vi "Autonomous Independent.vi"   [LabVIEW 2013]
doc: "This VI is called when autonomous begins, and will automatically be terminated when autonomous ends. You can carry out timed or sensor driven robot movement independently without needing to return to the caller."
uses:
  <vilib>/Rock Robotics/WPI/Solenoid/WPI_SolenoidValue.ctl
  Robot Global Data.vi
  <vilib>/Rock Robotics/WPI/Solenoid/WPI_SolenoidSetEnum.vi
  <vilib>/Rock Robotics/WPI/RobotDrive/WPI_RobotDriveArcadeDrive_Standard(NoSaturation).vi
  <vilib>/Rock Robotics/WPI/RobotDrive/WPI_RobotDriveGetSetRefNum.vi
  <vilib>/Rock Robotics/WPI/Joystick/WPI_JoystickGetSetRefNum.vi
panel:
  # "Be sure to right-click and choose Data Operations>>Make Current Value default if you want to save the array values with the VI"
types:
  T1 = typedef "WPI_JoystickDevRef.ctl" = cluster{"Device":T2}
  T2 = typedef "WPI_JoystickDeviceEnum.ctl" = enum16{"USB 1", "USB 2", "USB 3", "USB 4", "Kinect 1", "Kinect 2"}
  T3 = cluster{"axis 1 (x)":dbl, "axis 2 (y)":dbl, "axis 3 (throttle)":dbl, "axis 4":dbl, "axis 5":dbl, "axis 6":dbl}
  T4 = typedef "WPI_SolenoidValue.ctl" = enum16{"Off", "On", "Forward", "Reverse"}
  T5 = typedef "WPI_SolenoidDevRef.ctl" = cluster{"DevStatus":errorcluster, "Solenoid Module":T6, "Forward Solenoid Channel":T7, "Reverse Solenoid Channel":T7}
  T6 = typedef "FPGA_TypedefSolenoidModule.ctl" = enum16{"Solenoid Module 1", "Solenoid Module 2"}
  T7 = typedef "WPI_SolenoidChannel.ctl" = enum8{"Solenoid 1", "Solenoid 2", "Solenoid 3", "Solenoid 4", "Solenoid 5", "Solenoid 6", "Solenoid 7", "Solenoid 8", "Invalid"}
  T8 = typedef "WPI_RobotDriveDevRef.ctl" = cluster{"DevStatus":errorcluster, "Motors[]":T9[], "Square Inputs":bool, "Max Output":dbl, "Isochronous":bool}
  T9 = typedef "WPI_MotorControlDeviceRef.ctl" = cluster{"DeviceStatus":errorcluster, "Type":enum16{"PWM", "CAN"}, "PWM":cluster{"Digital Module":T10, "PWM Channel":T11, "DeadBand":T12}, "CAN":cluster{"Device Number":u8, "Control Mode":T13, "Semaphore":T14, "Max Vout":dbl}, "Invert":bool, "TransformRef":T15, "InvTransformRef":T15}
  T10 = typedef "FPGA_TypedefDigitalModule.ctl" = enum16{"Digital Module 1", "Digital Module 2"}
  T11 = typedef "FPGA_DIOPWMChannel.ctl" = enum8{"PWM 1", "PWM 2", "PWM 3", "PWM 4", "PWM 5", "PWM 6", "PWM 7", "PWM 8", "PWM 9", "PWM 10", "Invalid"}
  T12 = typedef "WPI_PWMDeadband.ctl" = cluster{"Name":string, "maxPositivePwm":i32, "minPositivePwm":i32, "centerPwm":i32, "maxNegativePwm":i32, "minNegativePwm":i32, "angularRange":u16}
  T13 = typedef "WPI_CANJaguar_ControlMode.ctl" = enum8{"Percent VBus", "Current", "Speed", "Position", "Voltage"}
  T14 = typedef "Semaphore RefNum" = refnum<k1>
  T15 = typedef "WPI_PWMTransform_ConPane.ctl" = refnum<vi>
  T16 = typedef "TargetType.ctl" = enum16{"Not Hot", "Hot"}
  T17 = cluster{"Distance (ft)":dbl, "Target Center (-1 to 1)":cluster{"X":dbl, "Y":dbl}, "Left":bool, "State":T16}[]
  T18 = cluster{"Distance (ft)":dbl, "Target Center (-1 to 1)":cluster{"X":dbl, "Y":dbl}, "Left":bool, "State":T16}
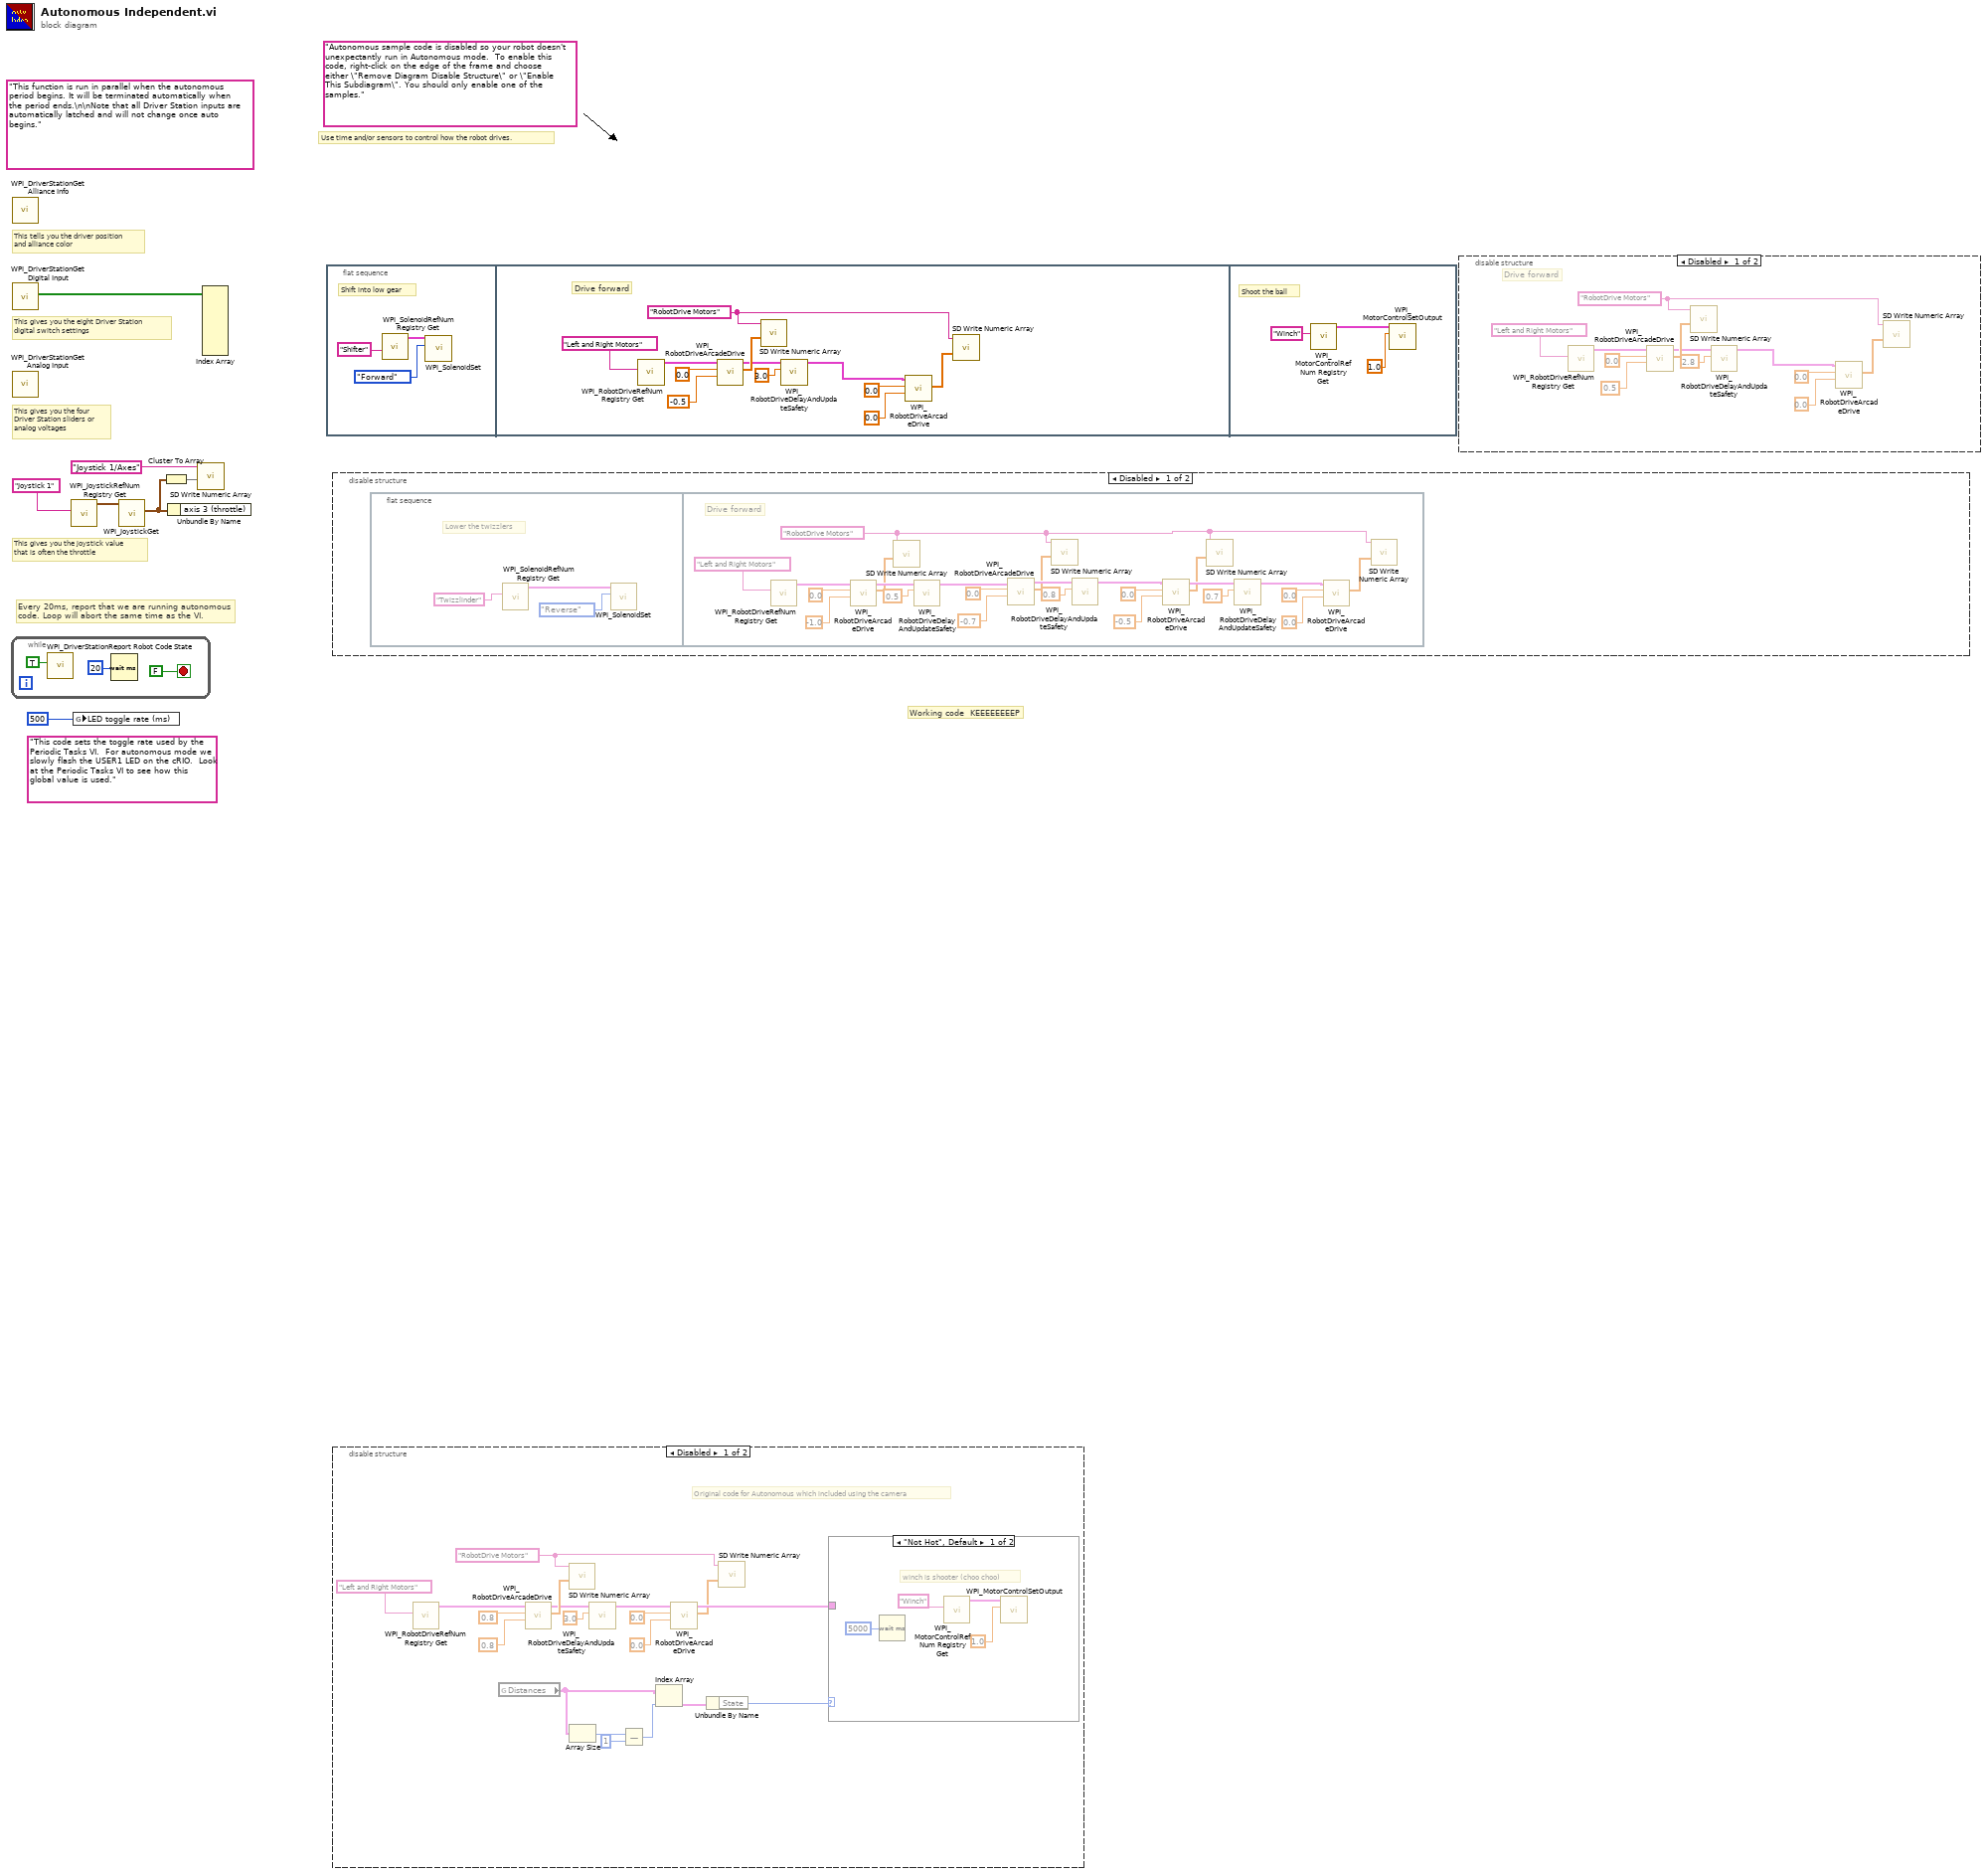
[diagram p0: block diagram]
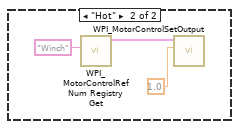
[diagram p4: hidden frame]
diagram:
  (unwired) "This code sets the toggle rate used by the Periodic Tasks VI.  For autonomous mode we slowly flash the USER1 LED on the cRIO.  Look at the Periodic Tasks VI to see how this global value is used."
  (unwired) "Autonomous sample code is disabled so your robot doesn't unexpectantly run in Autonomous mode.  To enable this code, right-click on the edge of the frame and choose either \"Remove Diagram Disable Structure\" or \"Enable This Subdiagram\". You should only enable one of the samples."
  (unwired) "This function is run in parallel when the autonomous period begins. It will be terminated automatically when the period ends.\n\nNote that all Driver Station inputs are automatically latched and will not change once auto begins."
  # "Working code  KEEEEEEEEP"
  # "Every 20ms, report that we are running autonomous\ncode. Loop will abort the same time as the VI."
  # "This gives you the joystick value\nthat is often the throttle"
  # "Use time and/or sensors to control how the robot drives."
  # "This tells you the driver position\nand alliance color"
  # "This gives you the eight Driver Station\ndigital switch settings"
  # "This gives you the four\nDriver Station sliders or\nanalog voltages"
  n1 = while {
    stop <- FALSE stop-if-true
    n2 = call <vilib>:"WPI_DriverStationReport Robot Code State.vi"("Autonomous"=TRUE) -> ()  [unwired: 10 in, 1 out]
    n3 = Wait (ms)(milliseconds to wait=u32 20) -> ()  [unwired: 1 out]
  }
  n4 = call <vilib>:"WPI_DriverStationGet Alliance Info.vi"() -> ()  [unwired: 12 out]
  n5 = call <vilib>:"WPI_DriverStationGet Digital Input.vi"() -> ("Driver Station Digital Input (1-8)"=w7:bool[])  [unwired: 11 out]
  n6 = call <vilib>:"WPI_DriverStationGet Analog Input.vi"() -> ()  [unwired: 12 out]
  n7 = call <vilib>:"WPI_JoystickRefNum Registry Get.vi"("refnum name"="Joystick 1") -> ("JoystickDevRef"=w5:T1)  [unwired: 1 in, 9 out]
  n8 = global write "Robot Global Data.vi" "LED toggle rate (ms)"(u32 500 ("LED ms toggle rate")) -> ()
  n9 = call <vilib>:"WPI_JoystickGet.vi"("JoystickDevRef"=w5) -> ("Axes"=w2:T3)  [unwired: 1 in, 5 out]
  n10 = Cluster To Array(cluster=w2) -> (array=w3:dbl[])
  n11 = Unbundle By Name(w2) -> ()  [unwired: 1 out]
  n12 = call <vilib>:"SD Write Numeric Array.vi"("Numeric Array"=w3, "Name"="Joystick 1/Axes") -> ()  [unwired: 8 in, 2 out]
  n13 = Index Array(array=w7) -> ()  [unwired: 8 in, 8 out]
  n14 = flat-sequence {
    frame #0 {
      # "Shift into low gear"
      n15 = call <vilib>:"WPI_SolenoidRefNum Registry Get.vi"("refnum name"="Shifter") -> ("SolenoidDevRef"=w12:T5)  [unwired: 9 in, 1 out]
      n16 = call-poly <vilib>:"WPI_SolenoidSet.vi"("Value"=WPI_SolenoidValue."Forward", "SolenoidDevRef"=w12) -> ()  [unwired: 1 in, 9 out]
    }
    frame #1 {
      w15 = "RobotDrive Motors" ("Name")
      # "Drive forward"
      n17 = call <vilib>:"WPI_RobotDriveRefNum Registry Get.vi"("refnum name"="Left and Right Motors") -> ("RobotDriveDevRef"=w24:T8)  [unwired: 1 in, 9 out]
      n18 = call-poly <vilib>:"WPI_RobotDriveArcadeDrive.vi"("Y axis value"=-0.5 ("X axis value"), "X axis value"=0.0, "RobotDriveDevRef"=w24) -> ("Motor Values"=w25:dbl[], "RobotDriveDevRef"=w21:T8)  [unwired: 1 in, 6 out]
      n19 = call <vilib>:"SD Write Numeric Array.vi"("Numeric Array"=w25, "Name"=w15) -> ()  [unwired: 8 in, 2 out]
      n20 = call <vilib>:"WPI_RobotDriveDelayAndUpdateSafety.vi"("Delay (s)"=3.0, "RobotDriveDevRef"=w21) -> ("RobotDriveDevRef 2"=w14:T8)  [unwired: 8 in, 1 out]
      n21 = call-poly <vilib>:"WPI_RobotDriveArcadeDrive.vi"("Y axis value"=0.0 ("X axis value"), "X axis value"=0.0, "RobotDriveDevRef"=w14) -> ("Motor Values"=w18:dbl[])  [unwired: 1 in, 7 out]
      n22 = call <vilib>:"SD Write Numeric Array.vi"("Numeric Array"=w18, "Name"=w15) -> ()  [unwired: 8 in, 2 out]
    }
    frame #2 {
      # "Shoot the ball"
      n23 = call <vilib>:"WPI_MotorControlRefNum Registry Get.vi"("refnum name"="Winch") -> ("MotorControlDevRef"=w27:T9)  [unwired: 9 in, 1 out]
      n24 = call <vilib>:"WPI_MotorControlSetOutput.vi"("Output"=1.0, "MotorControlDevRef"=w27) -> ()  [unwired: 7 in, 3 out]
    }
  }
  n25 = disable-structure shown="Disabled" {
    frame Disabled {
      n26 = flat-sequence {
        frame #0 {
          # "Lower the twizzlers"
          n27 = call <vilib>:"WPI_SolenoidRefNum Registry Get.vi"("refnum name"="Twizzlinder") -> ("SolenoidDevRef"=w30:T5)  [unwired: 9 in, 1 out]
          n28 = call-poly <vilib>:"WPI_SolenoidSet.vi"("Value"=WPI_SolenoidValue."Reverse", "SolenoidDevRef"=w30) -> ()  [unwired: 1 in, 9 out]
        }
        frame #1 {
          w55 = "RobotDrive Motors" ("Name")
          # "Drive forward"
          n29 = call <vilib>:"WPI_RobotDriveRefNum Registry Get.vi"("refnum name"="Left and Right Motors") -> ("RobotDriveDevRef"=w34:T8)  [unwired: 1 in, 9 out]
          n30 = call-poly <vilib>:"WPI_RobotDriveArcadeDrive.vi"("Y axis value"=-1.0 ("X axis value"), "X axis value"=0.0, "RobotDriveDevRef"=w34) -> ("Motor Values"=w33:dbl[], "RobotDriveDevRef"=w37:T8)  [unwired: 1 in, 6 out]
          n31 = call <vilib>:"SD Write Numeric Array.vi"("Numeric Array"=w33, "Name"=w55) -> ()  [unwired: 8 in, 2 out]
          n32 = call <vilib>:"WPI_RobotDriveDelayAndUpdateSafety.vi"("Delay (s)"=0.5, "RobotDriveDevRef"=w37) -> ("RobotDriveDevRef 2"=w47:T8)  [unwired: 8 in, 1 out]
          n33 = call-poly <vilib>:"WPI_RobotDriveArcadeDrive.vi"("Y axis value"=-0.7 ("X axis value"), "X axis value"=0.0, "RobotDriveDevRef"=w47) -> ("Motor Values"=w42:dbl[], "RobotDriveDevRef"=w44:T8)  [unwired: 1 in, 6 out]
          n34 = call <vilib>:"SD Write Numeric Array.vi"("Numeric Array"=w42, "Name"=w55) -> ()  [unwired: 8 in, 2 out]
          n35 = call <vilib>:"WPI_RobotDriveDelayAndUpdateSafety.vi"("Delay (s)"=0.8, "RobotDriveDevRef"=w44) -> ("RobotDriveDevRef 2"=w53:T8)  [unwired: 8 in, 1 out]
          n36 = call-poly <vilib>:"WPI_RobotDriveArcadeDrive.vi"("Y axis value"=-0.5 ("X axis value"), "X axis value"=0.0, "RobotDriveDevRef"=w53) -> ("Motor Values"=w48:dbl[], "RobotDriveDevRef"=w50:T8)  [unwired: 1 in, 6 out]
          n37 = call <vilib>:"SD Write Numeric Array.vi"("Numeric Array"=w48, "Name"=w55) -> ()  [unwired: 8 in, 2 out]
          n38 = call <vilib>:"WPI_RobotDriveDelayAndUpdateSafety.vi"("Delay (s)"=0.7, "RobotDriveDevRef"=w50) -> ("RobotDriveDevRef 2"=w54:T8)  [unwired: 8 in, 1 out]
          n39 = call-poly <vilib>:"WPI_RobotDriveArcadeDrive.vi"("Y axis value"=0.0 ("X axis value"), "X axis value"=0.0, "RobotDriveDevRef"=w54) -> ("Motor Values"=w32:dbl[])  [unwired: 1 in, 7 out]
          n40 = call <vilib>:"SD Write Numeric Array.vi"("Numeric Array"=w32, "Name"=w55) -> ()  [unwired: 8 in, 2 out]
        }
      }
    }
    frame Enabled {
    }
  }
  n41 = disable-structure shown="Disabled" {
    frame Disabled {
      w72 = "RobotDrive Motors" ("Name")
      # "Original code for Autonomous which included using the camera"
      n42 = call <vilib>:"WPI_RobotDriveRefNum Registry Get.vi"("refnum name"="Left and Right Motors") -> ("RobotDriveDevRef"=w69:T8)  [unwired: 1 in, 9 out]
      n43 = global read "Robot Global Data.vi" "Distances"() -> (w56:T17)
      n44 = call-poly <vilib>:"WPI_RobotDriveArcadeDrive.vi"("Y axis value"=0.8 ("X axis value"), "X axis value"=0.8, "RobotDriveDevRef"=w69) -> ("Motor Values"=w70:dbl[], "RobotDriveDevRef"=w66:T8)  [unwired: 1 in, 6 out]
      n45 = call <vilib>:"SD Write Numeric Array.vi"("Numeric Array"=w70, "Name"=w72) -> ()  [unwired: 8 in, 2 out]
      n46 = Array Size(array=w56) -> (size(s)=w57:i32)
      n47 = call <vilib>:"WPI_RobotDriveDelayAndUpdateSafety.vi"("Delay (s)"=3.0, "RobotDriveDevRef"=w66) -> ("RobotDriveDevRef 2"=w73:T8)  [unwired: 8 in, 1 out]
      n48 = Subtract(x=w57, y=1) -> (x-y=w59:i32)
      n49 = Index Array(array=w56, index=w59) -> (element=w60:T18)
      n50 = call-poly <vilib>:"WPI_RobotDriveArcadeDrive.vi"("Y axis value"=0.0 ("X axis value"), "X axis value"=0.0, "RobotDriveDevRef"=w73) -> ("Motor Values"=w71:dbl[], "RobotDriveDevRef"=w74:T8)  [unwired: 1 in, 6 out]
      n51 = Unbundle By Name(w60) -> ("State"=w61:T16)
      n52 = call <vilib>:"SD Write Numeric Array.vi"("Numeric Array"=w71, "Name"=w72) -> ()  [unwired: 8 in, 2 out]
      n53 = case shown="\"Not Hot\", Default" w61 {
        tunnel: w74 -> [_ _]
        frame "Not Hot", Default {
          # "winch is shooter (choo choo)"
          n54 = Wait (ms)(milliseconds to wait=u32 5000) -> ()  [unwired: 1 out]
          n55 = call <vilib>:"WPI_MotorControlRefNum Registry Get.vi"("refnum name"="Winch") -> ("MotorControlDevRef"=w76:T9)  [unwired: 9 in, 1 out]
          n56 = call <vilib>:"WPI_MotorControlSetOutput.vi"("Output"=1.0, "MotorControlDevRef"=w76) -> ()  [unwired: 7 in, 3 out]
        }
        frame "Hot" {
          n57 = call <vilib>:"WPI_MotorControlRefNum Registry Get.vi"("refnum name"="Winch") -> ("MotorControlDevRef"=w80:T9)  [unwired: 9 in, 1 out]
          n58 = call <vilib>:"WPI_MotorControlSetOutput.vi"("Output"=1.0, "MotorControlDevRef"=w80) -> ()  [unwired: 7 in, 3 out]
        }
      }
    }
    frame Enabled {
    }
  }
  n59 = disable-structure shown="Disabled" {
    frame Disabled {
      w83 = "RobotDrive Motors" ("Name")
      # "Drive forward"
      n60 = call <vilib>:"WPI_RobotDriveRefNum Registry Get.vi"("refnum name"="Left and Right Motors") -> ("RobotDriveDevRef"=w92:T8)  [unwired: 1 in, 9 out]
      n61 = call-poly <vilib>:"WPI_RobotDriveArcadeDrive.vi"("Y axis value"=0.5 ("X axis value"), "X axis value"=0.0, "RobotDriveDevRef"=w92) -> ("Motor Values"=w93:dbl[], "RobotDriveDevRef"=w89:T8)  [unwired: 1 in, 6 out]
      n62 = call <vilib>:"SD Write Numeric Array.vi"("Numeric Array"=w93, "Name"=w83) -> ()  [unwired: 8 in, 2 out]
      n63 = call <vilib>:"WPI_RobotDriveDelayAndUpdateSafety.vi"("Delay (s)"=2.8, "RobotDriveDevRef"=w89) -> ("RobotDriveDevRef 2"=w82:T8)  [unwired: 8 in, 1 out]
      n64 = call-poly <vilib>:"WPI_RobotDriveArcadeDrive.vi"("Y axis value"=0.0 ("X axis value"), "X axis value"=0.0, "RobotDriveDevRef"=w82) -> ("Motor Values"=w86:dbl[])  [unwired: 1 in, 7 out]
      n65 = call <vilib>:"SD Write Numeric Array.vi"("Numeric Array"=w86, "Name"=w83) -> ()  [unwired: 8 in, 2 out]
    }
    frame Enabled {
    }
  }
